vi "Drive_Simulated_Hardware.vi"() -> ()   [LabVIEW 2019]
uses:
  Subsystems/Drive/Drive_Globals.vi
  Subsystems/Sensing/Sensor_Values.vi
panel:
  out "XY Graph":cluster{"v_linear":dbl[], "v_linear":dbl[]}(graph)
  in  "Zero XY?":bool
  in  "k_magic":dbl
  in  "b_length":dbl
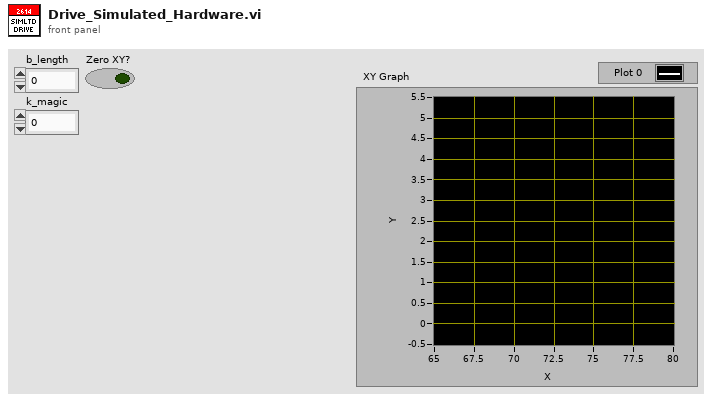
[diagram p1: front panel]
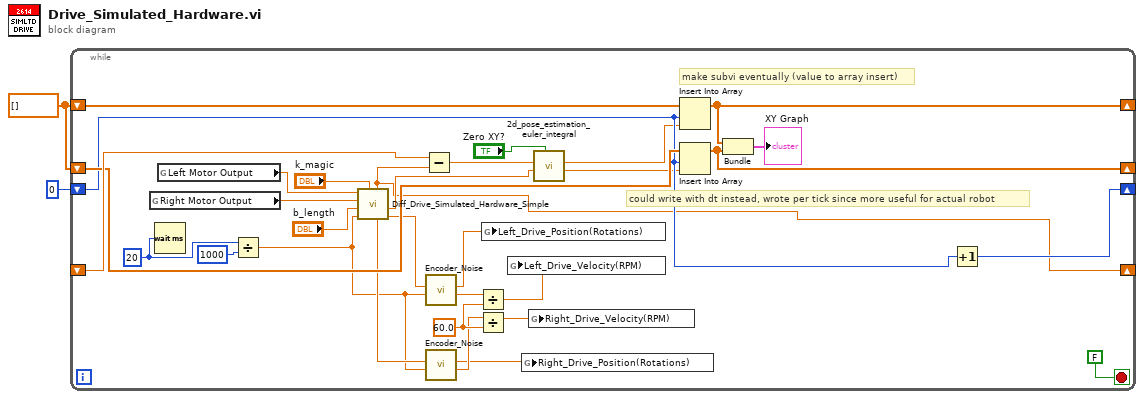
[diagram p0: block diagram]
diagram:
  w2 = dbl[] [] ("v_linear")
  n1 = while {
    shift-right: [w15] -> _
    shift-left: _ -> [w28]
    shift-right: [w17] -> _
    shift-left: w2 -> [w24]
    shift-right: [w16] -> _
    shift-left: w2 -> [w23]
    shift-right: [w21] -> _
    shift-left: u32 0 ("milliseconds to wait") -> [w22]
    stop <- FALSE stop-if-true
    w6 = 60.0 ("y")
    w32 = u32 20 ("milliseconds to wait")
    # "make subvi eventually (value to array insert)"
    # "could write with dt instead, wrote per tick since more useful for actual robot"
    n2 = global read "Drive_Globals.vi" "Right Motor Output"() -> (w13:dbl)
    n3 = Wait (ms)(milliseconds to wait=w32) -> ()  [unwired: 1 out]
    n4 = global read "Drive_Globals.vi" "Left Motor Output"() -> (w14:dbl)
    n5 = Divide(x=w32, y=u32 1000 ("milliseconds to wait")) -> (x/y=w10:dbl)
    n6 = call "Diff_Drive_Simulated_Hardware_Simple.vi"("k_magic"="k_magic", "delta_t"=w10, "b_length"="b_length", "%v_bus_right"=w13, "%v_bus_left"=w14) -> ("left_x"=w12:dbl, "x_angular"=w26:dbl, "right_x"=w11:dbl, "x_linear"=w15:dbl)  [unwired: 1 in, 2 out]
    n7 = Subtract(x=w28, y=w15) -> (x-y=w27:dbl)
    n8 = call "Encoder_Noise.vi"("dt(s)"=w10, "True Position(rotations)"=w12) -> ("Measured Velocity(rotations/sec)"=w9:dbl, "Measured Position(rotations)"=w7:dbl)  [unwired: 8 in]
    n9 = call "Encoder_Noise.vi"("dt(s)"=w10, "True Position(rotations)"=w11) -> ("Measured Velocity(rotations/sec)"=w5:dbl, "Measured Position(rotations)"=w3:dbl)  [unwired: 8 in]
    n10 = Divide(x=w9, y=w6) -> (x/y=w8:dbl)
    n11 = Divide(x=w5, y=w6) -> (x/y=w4:dbl)
    n12 = global write "Sensor_Values.vi" "Left_Drive_Position(Rotations)"(w7) -> ()
    n13 = global write "Sensor_Values.vi" "Left_Drive_Velocity(RPM)"(w8) -> ()
    n14 = global write "Sensor_Values.vi" "Right_Drive_Position(Rotations)"(w3) -> ()
    n15 = global write "Sensor_Values.vi" "Right_Drive_Velocity(RPM)"(w4) -> ()
    n16 = call "2d_pose_estimation_euler_integral.vi"("Zero XY?"="Zero XY?", "theta(rad)"=w26, "v(per tick)"=w27) -> ("y"=w19:dbl, "x"=w20:dbl)  [unwired: 7 in]
    n17 = Insert Into Array(array=w24, index=w22, new element=w20) -> (w17:dbl[])
    n18 = Insert Into Array(array=w23, index=w22, new element=w19) -> (w16:dbl[])
    n19 = Bundle("v_linear"=w17, "v_linear"=w16) -> (→"XY Graph":cluster{"v_linear":dbl[], "v_linear":dbl[]})  [unwired: 1 in]
    n20 = Increment(x=w22) -> (x+1=w21:u32)
  }
